vi "Alarmes.vi"() -> ()   [LabVIEW 2019]
panel:
  in  "Erro Rw":bool
  out "led Rw":bool
  out "aviso Rw":string
  in  "Erro Rk":bool
  out "led Rk":bool
  out "aviso Rk":string
  in  "Erro Vazio":bool
  out "led Vazio":bool
  out "aviso Vazio":string
  out "aviso SIT":string
  in  "Erro SIT":bool
  in  "stop":bool
  out "led SIT":bool
  in  "OK":bool
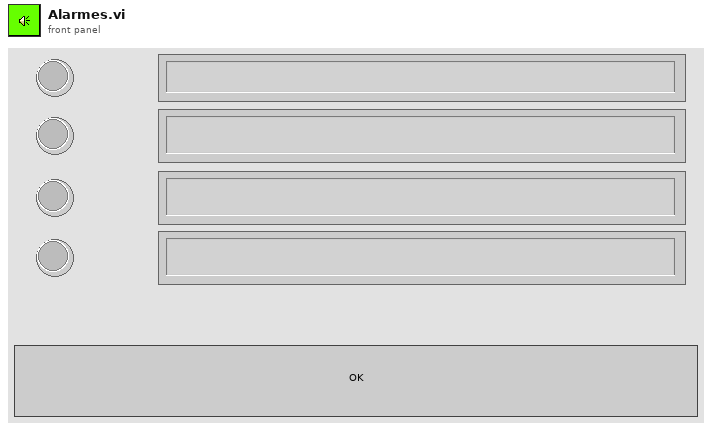
[diagram p1: front panel]
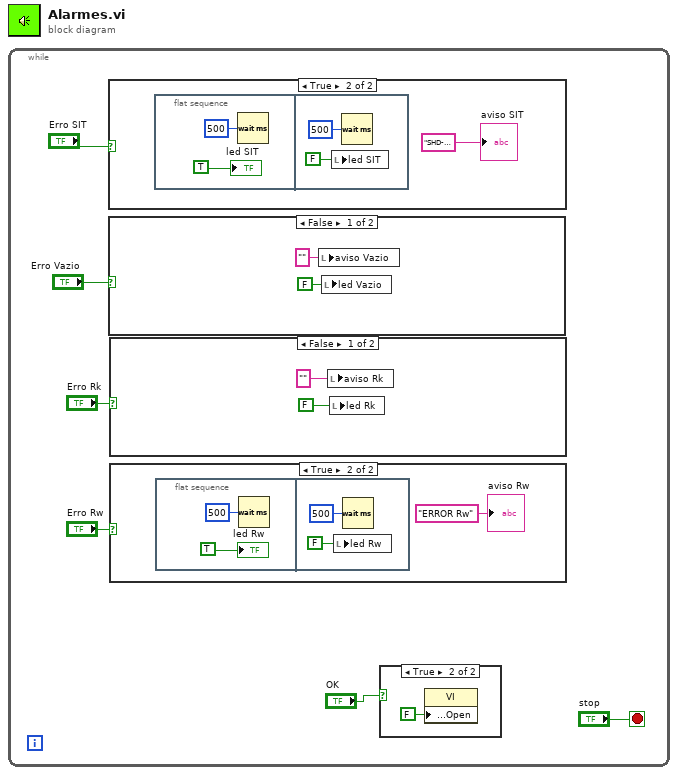
[diagram p0: block diagram]
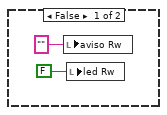
[diagram p2: hidden frame]
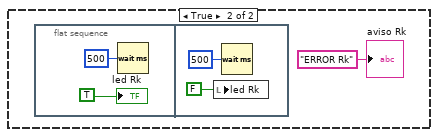
[diagram p3: hidden frame]
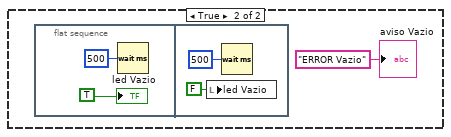
[diagram p4: hidden frame]
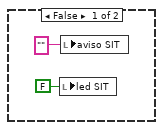
[diagram p5: hidden frame]
diagram:
  n1 = while {
    stop <- "stop" stop-if-true
    n2 = case shown="True" "Erro SIT" {
      frame False {
        n3 = local write "led SIT"(FALSE ("led SIT")) -> ()
        n4 = local write "aviso SIT"("" ("String")) -> ()
      }
      frame True {
        n5 = flat-sequence {
          frame #0 {
            n6 = Wait (ms)(milliseconds to wait=u32 500) -> ()  [unwired: 1 out]
            "led SIT" <- TRUE ("Boolean")
          }
          frame #1 {
            n7 = local write "led SIT"(FALSE ("Erro SIT")) -> ()
            n8 = Wait (ms)(milliseconds to wait=u32 500) -> ()  [unwired: 1 out]
          }
        }
        "aviso SIT" <- "SHD-PI-XX ATENÇÃO: DIFERENÇA ENTRE SHD-PI-01 E SHD-PI-02 MAIOR QUE 5%!!!" ("String")
      }
    }
    n9 = case shown="False" "Erro Vazio" {
      frame False {
        n10 = local write "aviso Vazio"("" ("aviso Vazio")) -> ()
        n11 = local write "led Vazio"(FALSE ("led Vazio")) -> ()
      }
      frame True {
        n12 = flat-sequence {
          frame #0 {
            n13 = Wait (ms)(milliseconds to wait=u32 500) -> ()  [unwired: 1 out]
            "led Vazio" <- TRUE ("Boolean")
          }
          frame #1 {
            n14 = local write "led Vazio"(FALSE ("Erro SIT")) -> ()
            n15 = Wait (ms)(milliseconds to wait=u32 500) -> ()  [unwired: 1 out]
          }
        }
        "aviso Vazio" <- "ERROR Vazio" ("String")
      }
    }
    n16 = case shown="False" "Erro Rk" {
      frame False {
        n17 = local write "aviso Rk"("" ("aviso Vazio")) -> ()
        n18 = local write "led Rk"(FALSE ("led Vazio")) -> ()
      }
      frame True {
        n19 = flat-sequence {
          frame #0 {
            n20 = Wait (ms)(milliseconds to wait=u32 500) -> ()  [unwired: 1 out]
            "led Rk" <- TRUE ("Boolean")
          }
          frame #1 {
            n21 = local write "led Rk"(FALSE ("Erro SIT")) -> ()
            n22 = Wait (ms)(milliseconds to wait=u32 500) -> ()  [unwired: 1 out]
          }
        }
        "aviso Rk" <- "ERROR Rk" ("String")
      }
    }
    n23 = case shown="True" "Erro Rw" {
      frame False {
        n24 = local write "aviso Rw"("" ("aviso Vazio")) -> ()
        n25 = local write "led Rw"(FALSE ("led Vazio")) -> ()
      }
      frame True {
        n26 = flat-sequence {
          frame #0 {
            n27 = Wait (ms)(milliseconds to wait=u32 500) -> ()  [unwired: 1 out]
            "led Rw" <- TRUE ("Boolean")
          }
          frame #1 {
            n28 = local write "led Rw"(FALSE ("Erro SIT")) -> ()
            n29 = Wait (ms)(milliseconds to wait=u32 500) -> ()  [unwired: 1 out]
          }
        }
        "aviso Rw" <- "ERROR Rw" ("String")
      }
    }
    n30 = case shown="True" "OK" {
      frame False {
      }
      frame True {
        n31 = property class="VI"("Front Panel.Open"=FALSE ("Front Panel Window:Open")) -> ()  [unwired: 2 in, 2 out]
      }
    }
  }
